vi "spring - add item.vi"(6 "new indentation":i32=-1, 7 "tree ref":refnum<vi>, 8 "error in (no error)":errorcluster, 9 "position (0=just below parent etc.)":i32, 10 "parent tag":string, 11 "itemstrings":string[](array[string])) -> (0 "error out":errorcluster, 3 "node data out":T1)   [LabVIEW 2014]
uses:
  spring - node data.ctl
panel:
  in  "node data typedef":T1
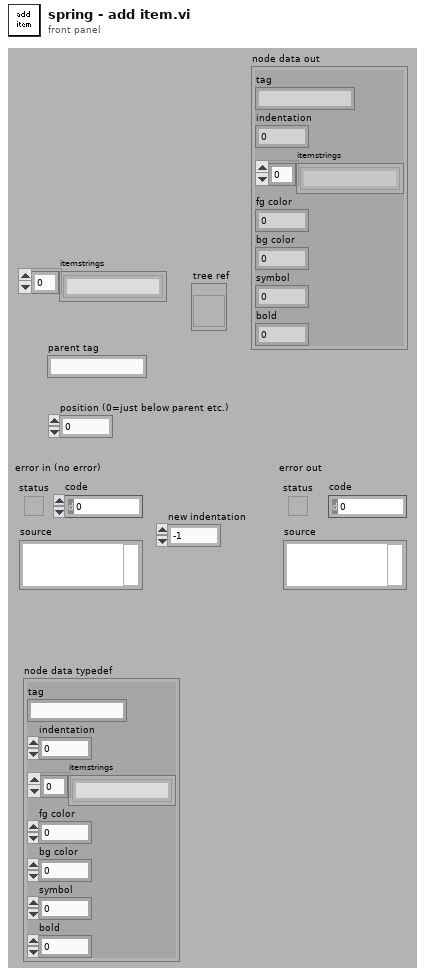
[diagram p1: front panel]
types:
  T1 = typedef "spring - node data.ctl" = cluster{"tag":string, "indentation":i32, "itemstrings":string[], "fg color":u32, "bg color":u32, "symbol":u32, "bold":u32}
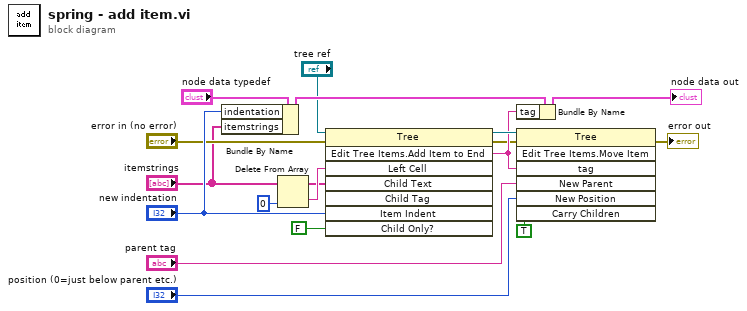
[diagram p0: block diagram]
diagram:
  n1 = Bundle By Name(cluster="node data typedef", "indentation"="new indentation", "itemstrings"="itemstrings") -> (w12:T1)
  n2 = Delete From Array(array="itemstrings", index=0) -> (deleted portion=w9:string, array with subset deleted=w8:string[])  [unwired: 1 in]
  n3 = invoke class="Tree" method="Edit Tree Items.Add Item to End"(reference="tree ref", error in="error in (no error)", "Left Cell"=w9, "Child Text"=w8, "Item Indent"="new indentation", "Child Only?"=FALSE) -> (reference out=w10:refnum<vi>, error out=w4:errorcluster, "Edit Tree Items:Add Item to End"=w5:string)  [unwired: 2 in, 5 out]
  n4 = Bundle By Name(cluster=w12, "tag"=w5) -> (→"node data out":T1)
  n5 = invoke class="Tree" method="Edit Tree Items.Move Item"(reference=w10, error in=w4, "tag"=w5, "New Parent"="parent tag", "New Position"="position (0=just below parent etc.)", "Carry Children"=TRUE) -> (error out=→"error out":errorcluster)  [unwired: 1 in, 6 out]
